vi "Set_Parameter_Instrument (Json).vi"(8 "error in (no error)":errorcluster caption="entrée d'erreur (pas d'erreur)", 10 "Parameter (Json)":string, 11 "Disable_DIO en entrée":refnum<class "Disable_DIO.lvclass">) -> (0 "error out":errorcluster caption="sortie d'erreur", 3 "Disable_DIO en sortie":refnum<class "Disable_DIO.lvclass">)   [LabVIEW 2020, in "Library Test.lvlib" / "Disable_DIO.lvclass"]
uses:
  Disable_DIO.lvclass
  C:/Users/ngarcin/OneDrive - Altyor/Standard TB/Class/Test/Test (Default)/Test (Default).lvclass
  Commun VI/TypeDef/Commande DIO/Parameter DIO.ctl
  DIO/Class DIO (Default)/Class DIO (Default).lvclass
  JSON API/JSON Value/Set from JSON string.vi
  JSON API/Variant JSON/Variant to JSON.vi
  JSON API/JSON Value/Get Item by name array.vi
  Test_Wtih_Instr/Test_With_Inst.lvclass
  Instrument/Instrument (Default)/Class Instrument (Default).lvclass
  JSON API/JSON Value/JSON Value.lvclass
  Disable_DIO.lvclass/Disable_DIO.ctl
  JSON API/Variant JSON/Variant JSON.lvlib
  JSON API/Get Polymorphic/JSON GetSet.lvlib
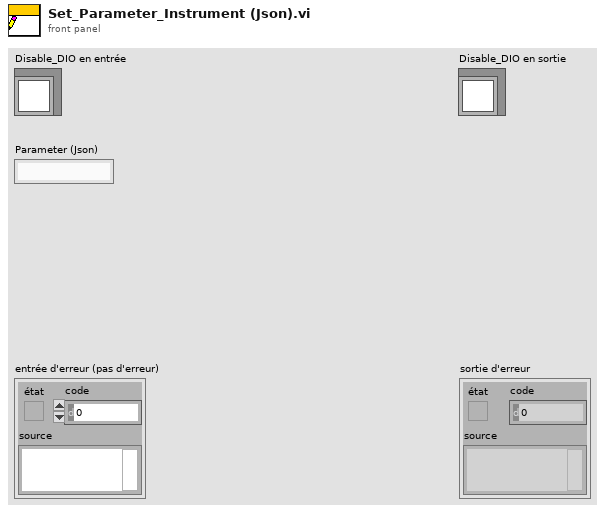
[diagram p1: front panel]
types:
  T1 = typedef "Parameter DIO.ctl" = cluster{"Device_Com_Port":string, "Port":u8, "Line":u8, "Function":enum16{"Write", "Read"}, "Class DIO":refnum<class "Class DIO (Default).lvclass">}
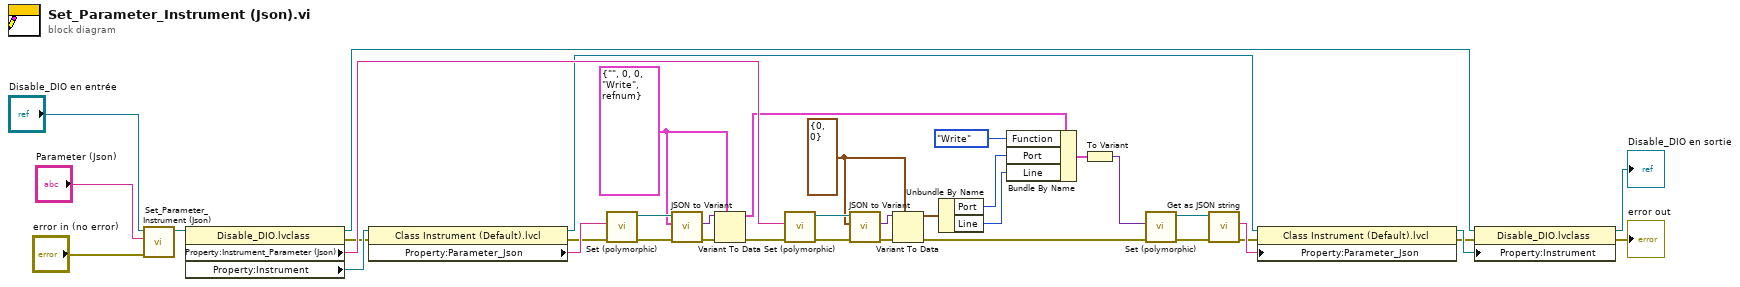
[diagram p0: block diagram]
diagram:
  w18 = T1 {"Device_Com_Port"="", "Port"=0, "Line"=0, "Function"=enum."Write", "Class DIO"=refnum} ("Parameter")
  w17 = cluster{"Line":u8, "Port":u8} {"Line"=0, "Port"=0} ("Cluster des données privées de classe")
  n1 = call-parent "Set_Parameter_Instrument (Json).vi"("error in (no error)"="error in (no error)", "Parameter (Json)"="Parameter (Json)", "Test (Default) en entrée"="Disable_DIO en entrée") -> ("Test (Default) en sortie"=w24:refnum<class "Disable_DIO.lvclass">)  [unwired: 7 in, 1 out]
  n2 = property class="Disable_DIO.lvclass"(reference=w24) -> (reference out=w20:refnum<class "Disable_DIO.lvclass">, error out=w5:errorcluster, "Property:Instrument_Parameter (Json)"=w22:string, "Property:Instrument"=w23:refnum<class "Class Instrument (Default).lvclass">)  [unwired: 1 in]
  n3 = property class="Class Instrument (Default).lvcl"(reference=w23, error in=w5) -> (reference out=w19:refnum<class "Class Instrument (Default).lvclass">, error out=w28:errorcluster, "Property:Parameter_Json"=w30:string)
  n4 = call-poly "Set (polymorphic).vi"("error in (no error)"=w28, "JSON stream"=w30) -> ("error out"=w32:errorcluster, "JSON Value out"=w34:refnum<class "JSON Value.lvclass">)  [unwired: 7 in, 1 out]
  n5 = call "JSON to Variant.vi"("error in (no error)"=w32, "Variant (Data Type)"=w18, "JSON Value"=w34) -> ("error out"=w33:errorcluster, "Variant out"=w31:variant)  [unwired: 7 in]
  n6 = Variant To Data(error in=w33, type=w18, Variant=w31) -> (data=w16:T1, error out=w29:errorcluster)
  n7 = call-poly "Set (polymorphic).vi"("error in (no error)"=w29, "JSON stream"=w22) -> ("error out"=w37:errorcluster, "JSON Value out"=w35:refnum<class "JSON Value.lvclass">)  [unwired: 7 in, 1 out]
  n8 = call "JSON to Variant.vi"("error in (no error)"=w37, "Variant (Data Type)"=w17, "JSON Value"=w35) -> ("error out"=w36:errorcluster, "Variant out"=w38:variant)  [unwired: 7 in]
  n9 = Variant To Data(error in=w36, type=w17, Variant=w38) -> (data=w14:cluster{"Line":u8, "Port":u8}, error out=w4:errorcluster)
  n10 = Unbundle By Name(w14) -> ("Port"=w13:u8, "Line"=w12:u8)
  n11 = Bundle By Name(cluster=w16, "Function"=enum16{"Write", "Read"}."Write", "Port"=w13, "Line"=w12) -> (w15:T1)
  n12 = To Variant(anything=w15) -> (Variant=w26:variant)
  n13 = call-poly "Set (polymorphic).vi"("error in (no error)"=w4, "Variant"=w26) -> ("error out"=w3:errorcluster, "JSON Value out"=w27:refnum<class "JSON Value.lvclass">)  [unwired: 8 in]
  n14 = call "Get as JSON string.vi"("error in (no error)"=w3, "JSON Value in"=w27) -> ("error out"=w2:errorcluster, "<JSON>"=w25:string)  [unwired: 8 in]
  n15 = property class="Class Instrument (Default).lvcl"(reference=w19, error in=w2, "Property:Parameter_Json"=w25) -> (reference out=w21:refnum<class "Class Instrument (Default).lvclass">, error out=w1:errorcluster)
  n16 = property class="Disable_DIO.lvclass"(reference=w20, error in=w1, "Property:Instrument"=w21) -> (reference out=→"Disable_DIO en sortie":refnum<class "Disable_DIO.lvclass">, error out=→"error out":errorcluster)
